vi "Complex to Polar Waveform.vi"(0 "Input Signal":waveform(cdb)) -> (1 "Angle":waveform(dbl), 2 "Magnitude":waveform(dbl))   [LabVIEW 2020]
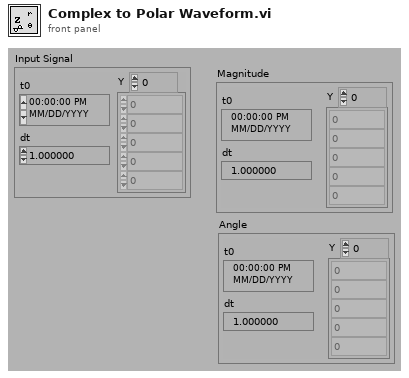
[diagram p1: front panel]
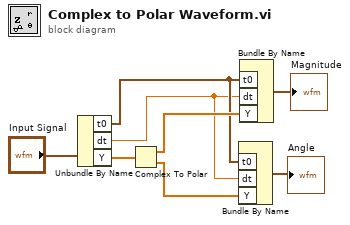
[diagram p0: block diagram]
diagram:
  n1 = Unbundle By Name("Input Signal") -> ("t0"=w4:timestamp, "dt"=w3:dbl, "Y"=w7:cdb[])
  n2 = Complex To Polar(r * e^(i*theta)=w7) -> (r=w6:dbl[], theta=w5:dbl[])
  n3 = Bundle By Name("t0"=w4, "dt"=w3, "Y"=w5) -> (→"Angle":waveform(dbl))  [unwired: 1 in]
  n4 = Bundle By Name("t0"=w4, "dt"=w3, "Y"=w6) -> (→"Magnitude":waveform(dbl))  [unwired: 1 in]
